vi "Is TLS.vi"(8 "error in (no error)":errorcluster, 11 "TCP Stream in":refnum<class "TCP Stream.lvclass">) -> (0 "error out":errorcluster, 2 "TLS?":bool, 3 "TCP Stream out":refnum<class "TCP Stream.lvclass">)   [LabVIEW 2024, in "Stream-TCP.lvlib" / "TCP Stream.lvclass"]
uses:
  TCP Stream.lvclass
  TCP Stream.lvclass/TCP Stream.ctl
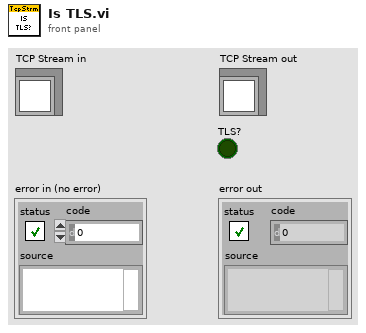
[diagram p1: front panel]
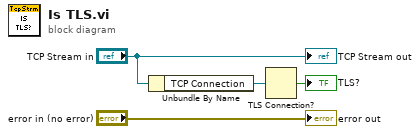
[diagram p0: block diagram]
diagram:
  n1 = Unbundle By Name("TCP Stream in") -> ("TCP Connection"=w2:refnum<k5>)
  n2 = TLS Connection?(1:w2) -> (0:→"TLS?":bool)
  "error out" <- "error in (no error)"
  "TCP Stream out" <- "TCP Stream in"
